vi "Sequence.UpdateMainTask.vi"(8 "error in (no error)":errorcluster, 11 "Refs":T1) -> (0 "error out":errorcluster, 3 "Task.Main Ref":refnum<k24>)   [LabVIEW 2013, in "Simple Sequence Tools - Editor.lvlib"]
uses:
  Simple Sequence Tools - Editor.lvlib
  Types/Sequence.MainSeqRefs.ctl
  NationalInstruments.VeriStand.RealTimeSequenceDefinitionApi
  Shared/SubVIs/Constants.vi
  Shared/Simple Sequence Tools - Shared.lvlib
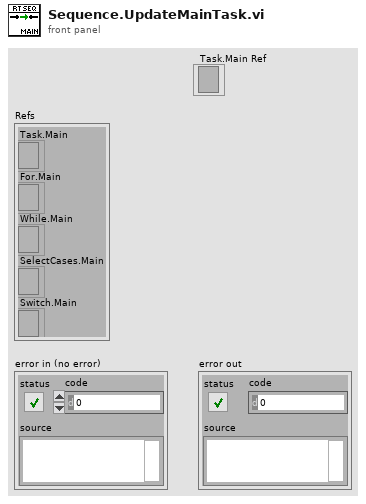
[diagram p1: front panel]
types:
  T1 = typedef "Simple Sequence Tools - Editor.lvlib/Sequence.MainSeqRefs.ctl" = cluster{"Task.Main":refnum<k24>, "For.Main":refnum<k24>, "While.Main":refnum<k24>, "SelectCases.Main":refnum<k24>, "Switch.Main":refnum<k24>}
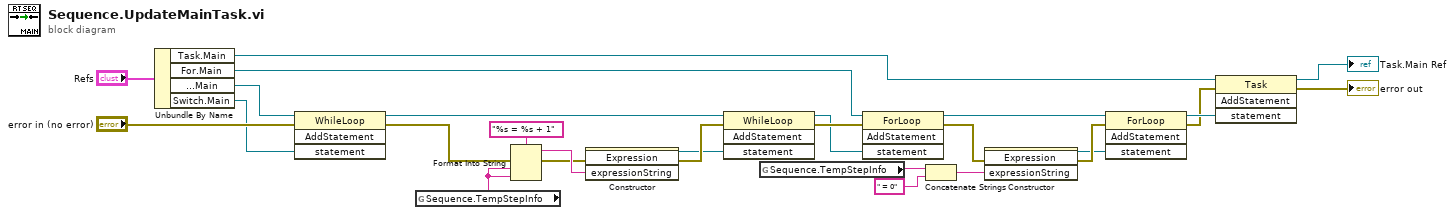
[diagram p0: block diagram]
diagram:
  n1 = Unbundle By Name("Refs") -> ("Task.Main"=w24:refnum<k24>, "For.Main"=w23:refnum<k24>, "While.Main"=w17:refnum<k24>, "Switch.Main"=w1:refnum<k24>)
  n2 = invoke class="WhileLoop" method="AddStatement"(reference=w17, error in="error in (no error)", "statement"=w1) -> (reference out=w9:refnum<k24>, error out=w18:errorcluster)  [unwired: 1 in, 2 out]
  n3 = global read "Constants.vi" "Sequence.TempStepInfo"() -> (w21:string)
  n4 = Format Into String(format string="%s = %s + 1" ("expressionString"), error in=w18, w21, w21) -> (resulting string=w22:string, error out=w19:errorcluster)  [unwired: 1 in]
  n5 = constructor class="Expression"(error in=w19, "expressionString"=w22) -> (reference out=w8:refnum<k24>, error out=w10:errorcluster)  [unwired: 2 in, 2 out]
  n6 = invoke class="WhileLoop" method="AddStatement"(reference=w9, error in=w10, "statement"=w8) -> (reference out=w11:refnum<k24>, error out=w12:errorcluster)  [unwired: 1 in, 2 out]
  n7 = global read "Constants.vi" "Sequence.TempStepInfo"() -> (w25:string)
  n8 = invoke class="ForLoop" method="AddStatement"(reference=w23, error in=w12, "statement"=w11) -> (reference out=w3:refnum<k24>, error out=w6:errorcluster)  [unwired: 1 in, 2 out]
  n9 = Concatenate Strings(w25, " = 0" ("string")) -> (w27:string)
  n10 = constructor class="Expression"(error in=w6, "expressionString"=w27) -> (reference out=w5:refnum<k24>, error out=w7:errorcluster)  [unwired: 2 in, 2 out]
  n11 = invoke class="ForLoop" method="AddStatement"(reference=w3, error in=w7, "statement"=w5) -> (reference out=w4:refnum<k24>, error out=w2:errorcluster)  [unwired: 1 in, 2 out]
  n12 = invoke class="Task" method="AddStatement"(reference=w24, error in=w2, "statement"=w4) -> (reference out=→"Task.Main Ref":refnum<k24>, error out=→"error out":errorcluster)  [unwired: 1 in, 2 out]
